vi "Write Run_Time.vi"(8 "error in (no error)":errorcluster, 10 "Run_Time":refnum<vi>, 11 "Chronometer in":refnum<class "Chronometer.lvclass">) -> (0 "error out":errorcluster, 3 "Chronometer out":refnum<class "Chronometer.lvclass">)   [LabVIEW 2023, in "Chronometer.lvlib" / "Chronometer.lvclass"]
uses:
  Chronometer.lvclass
  Chronometer.lvclass/Chronometer.ctl
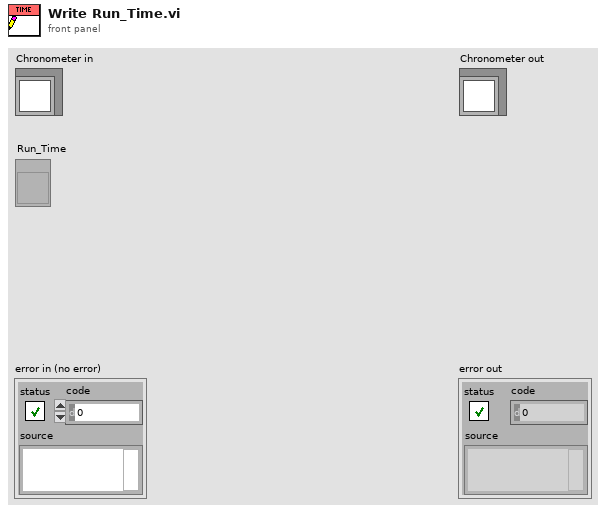
[diagram p1: front panel]
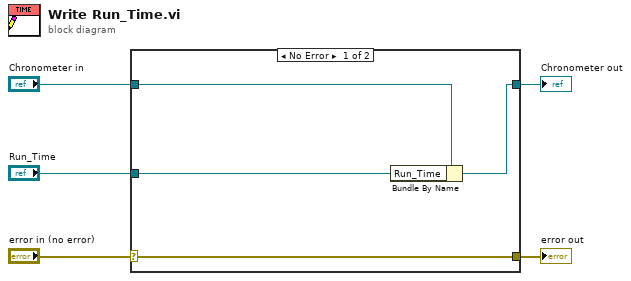
[diagram p0: block diagram]
diagram:
  n1 = case shown="No Error" "error in (no error)" {
    selector: "error in (no error)" -> [w9 w10]
    tunnel: [w9 w10] -> w4
    tunnel: [w7 w11] -> w2
    tunnel: "Chronometer in" -> [w8 w11]
    tunnel: "Run_Time" -> [w6 _]
    frame No Error {
      n2 = Bundle By Name(cluster=w8, "Run_Time"=w6) -> (w7:refnum<class "Chronometer.lvclass">)
    }
    frame Error {
    }
  }
  "error out" <- w4
  "Chronometer out" <- w2
